vi "webqq.vi"(2 "获取好友列表按钮":bool, 3 "确定按钮":bool, 5 "退出登录按钮":bool, 6 "发送按钮":bool, 7 "要发送的内容":string, 10 "确认搜索按钮":bool, 11 "输入QQ昵称":string) -> (4 "发送返回值":string, 8 "获取好友标志":bool, 9 "搜索出的对应ID":string)   [LabVIEW 2016]
uses:
  <vilib>/httpClient/LabVIEWHTTPClient.lvlib
panel:
  out "链接标志":bool
  out "qqbat字符串":string
  out "昵称对应ID":string[](array[string])
  out "图片路径":path
  out "QQ昵称":string[](array[string])
  out "ID":i32[](array[numeric])
  out "数值":dbl
  out "error out 2":errorcluster caption="错误输出"
  out "好友列表字符串":string
  in  "id":string
  out "QQ登录二维码":picture
  out "路径 2":path
  out "error out":errorcluster caption="错误输出"
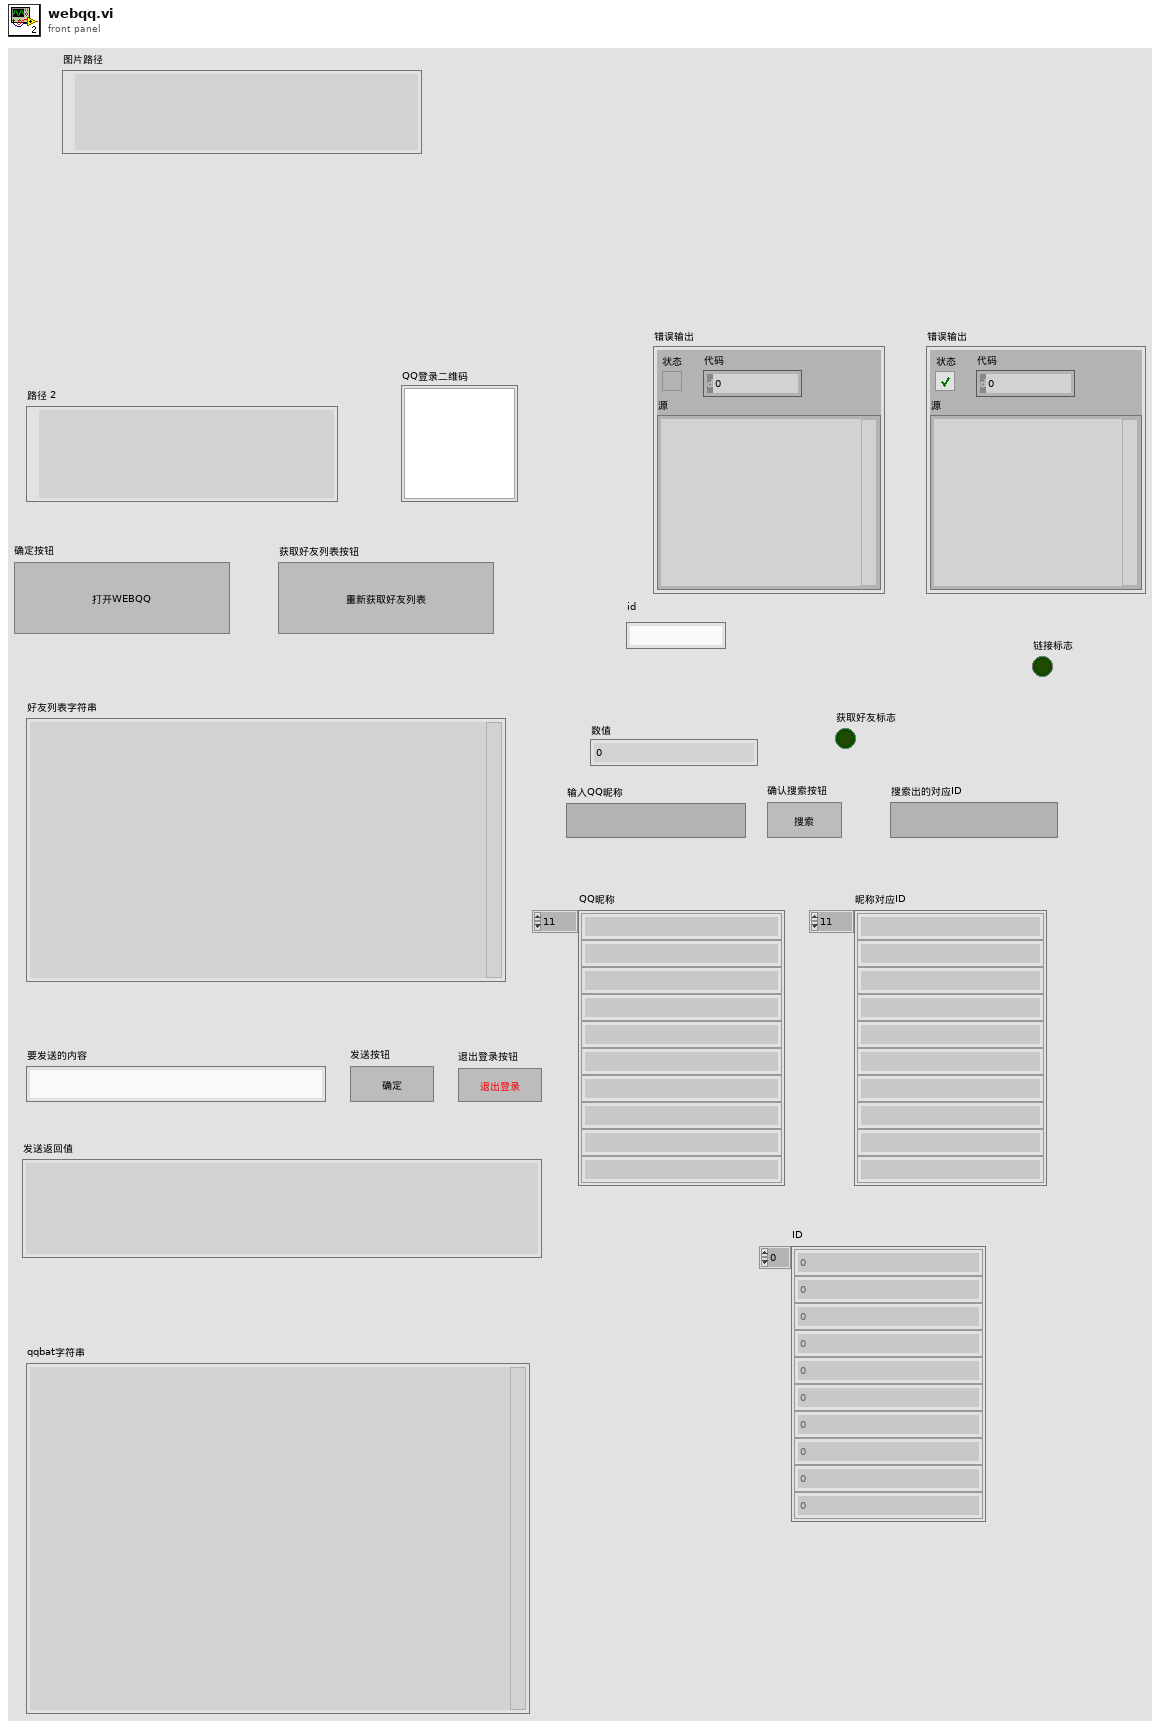
[diagram p1: front panel]
types:
  T1 = enum8{"Enabled", "Disabled", "Disabled and Grayed Out"}
  T2 = typedef "imagedata.ctl" = cluster{"image type":i32, "image depth":i32, "image":u8[], "mask":u8[], "colors":u32[], "Rectangle":cluster{"left":i16, "top":i16, "right":i16, "bottom":i16}}
  T3 = typedef "LabVIEWHTTPClient.lvlib/ClientHandle.ctl" = refnum<k1>
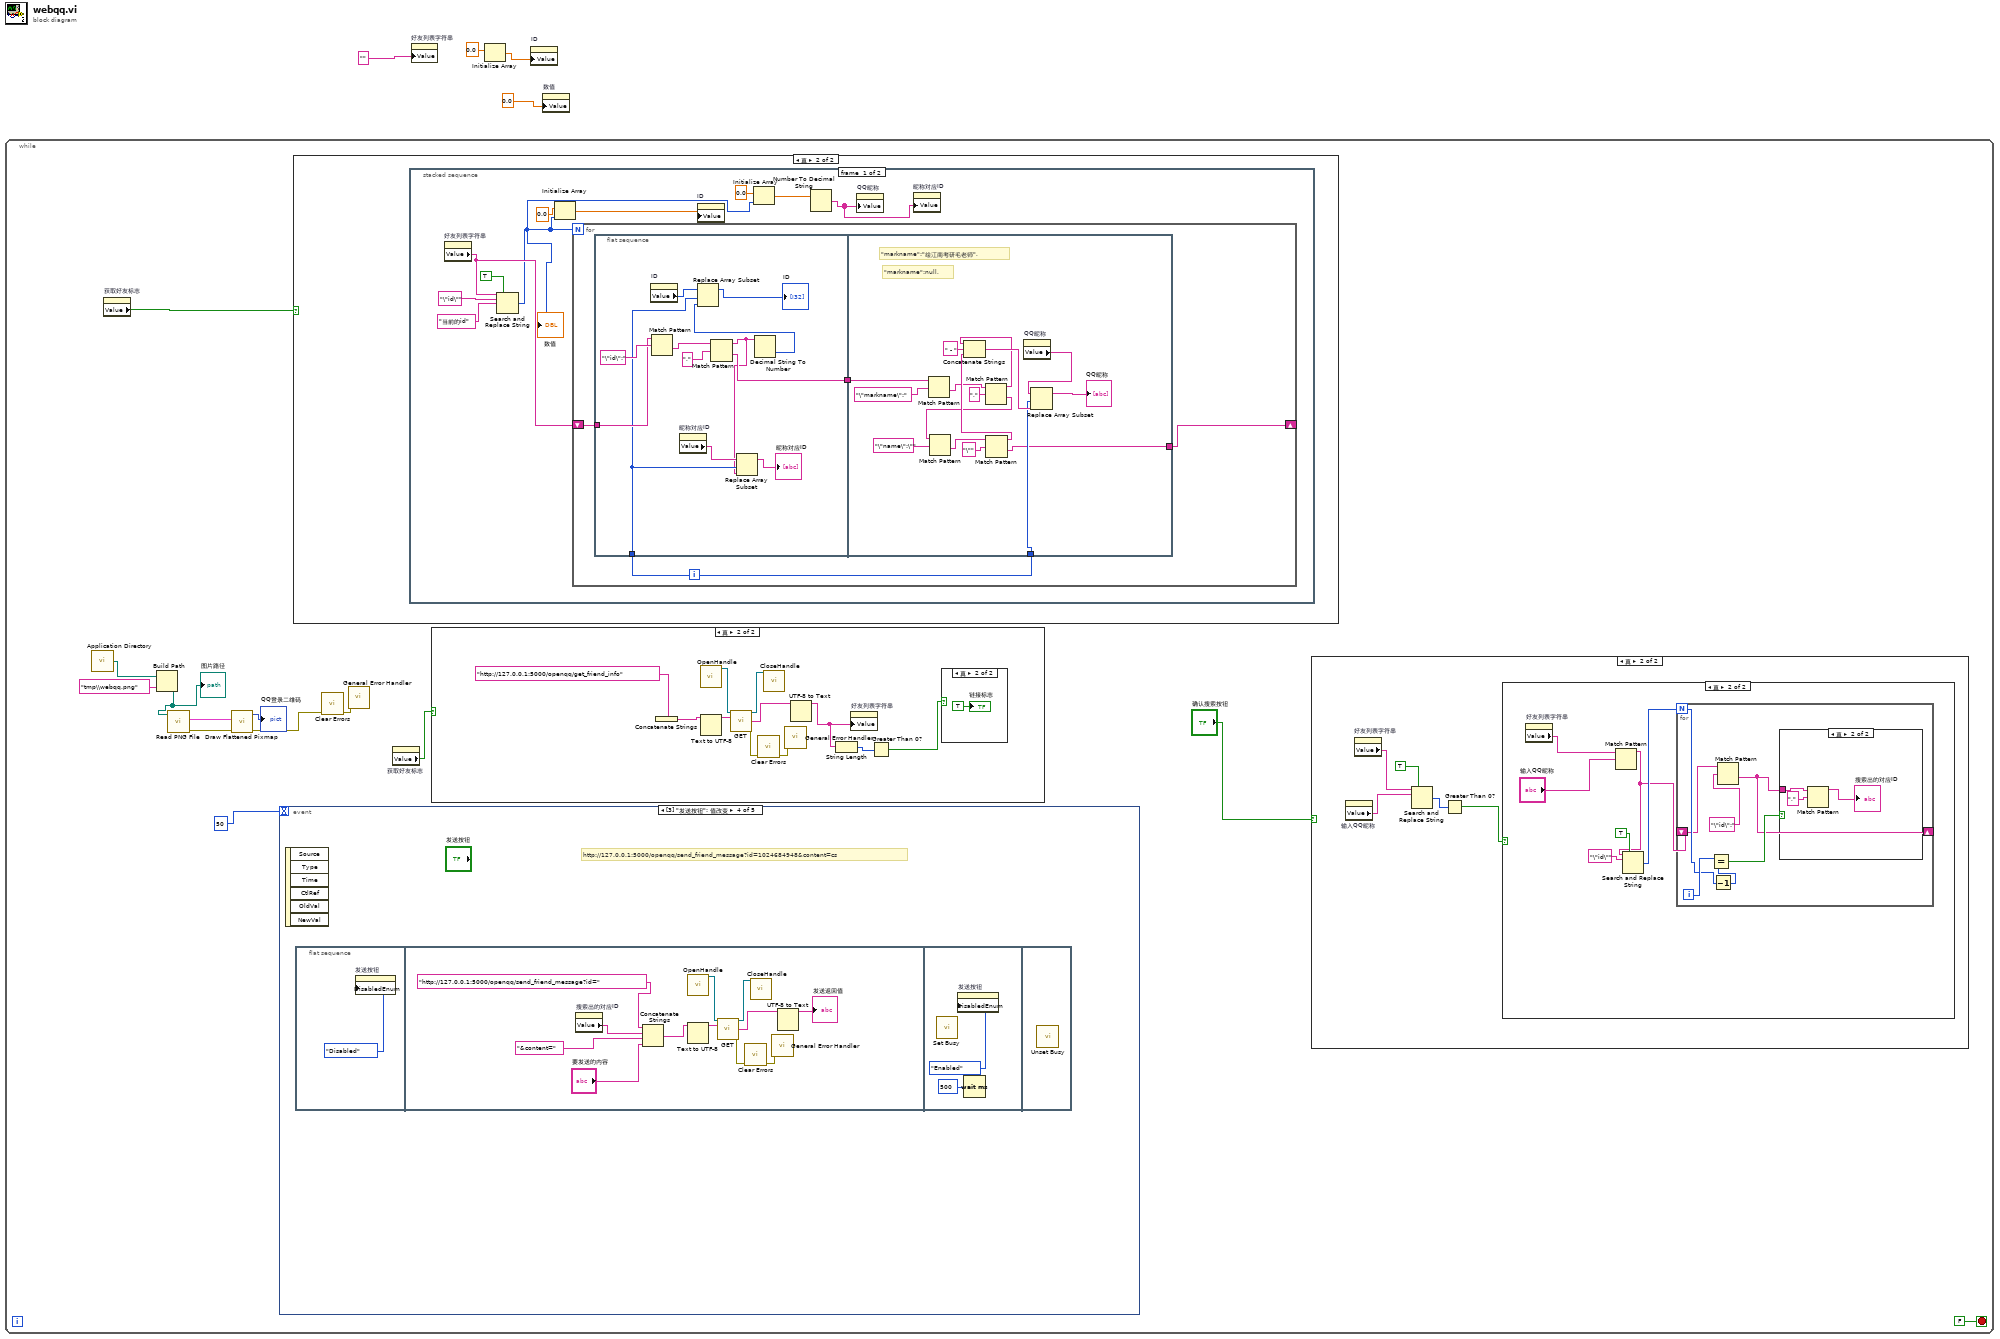
[diagram p0: block diagram]
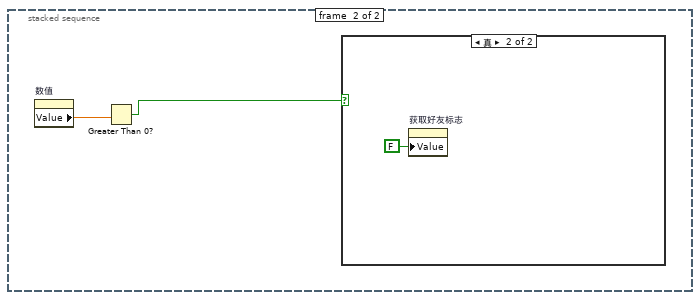
[diagram p8: hidden frame]
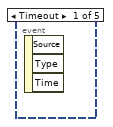
[diagram p10: hidden frame]
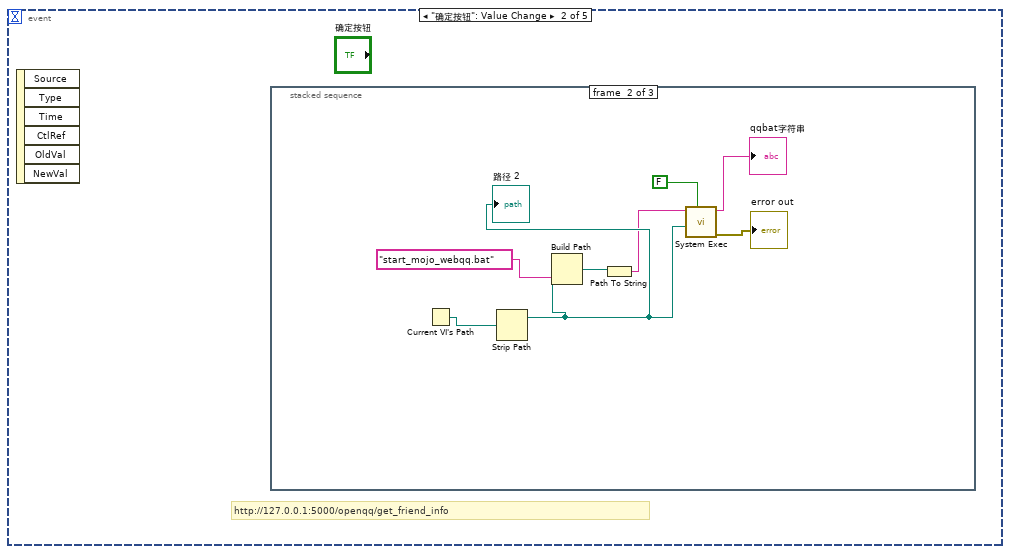
[diagram p11: hidden frame]
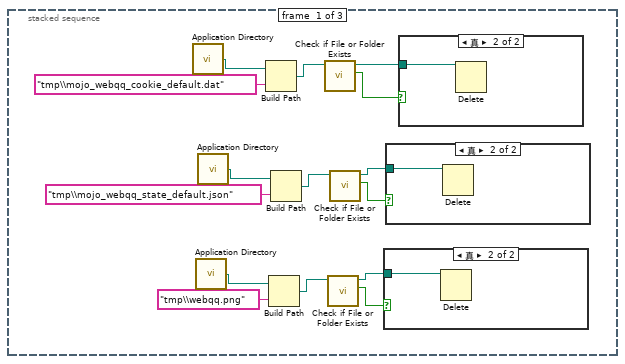
[diagram p12: hidden frame]
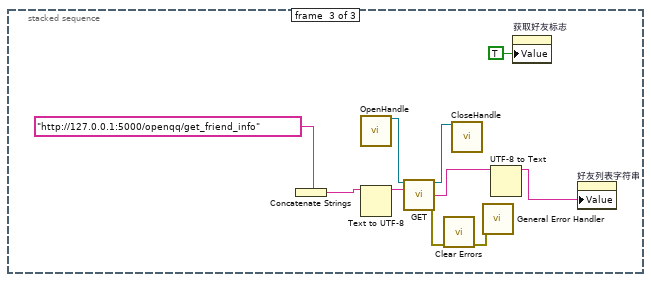
[diagram p16: hidden frame]
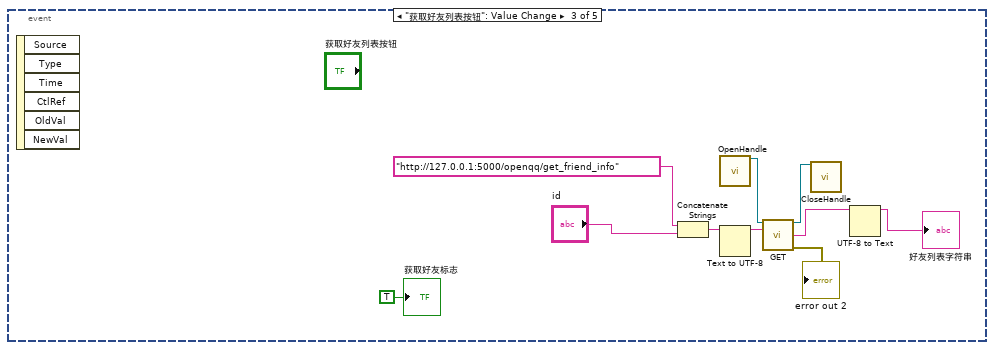
[diagram p17: hidden frame]
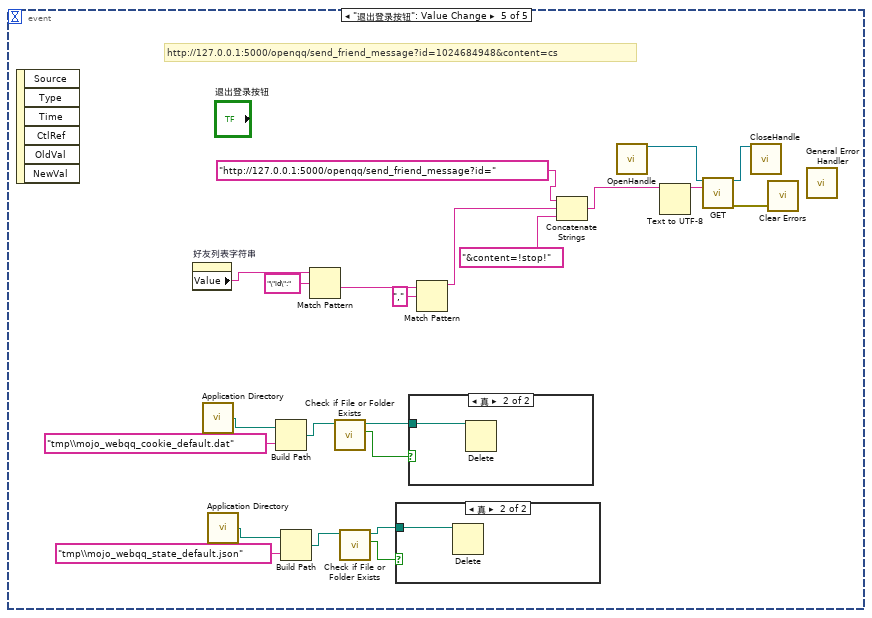
[diagram p18: hidden frame]
diagram:
  n1 = while {
    stop <- FALSE stop-if-true
    n2 = call <vilib>:"Application Directory.vi"() -> ("Application Directory"=w10:path)
    n3 = property on="获取好友标志" class="Bool (严格)"() -> ("Value"=w12:bool)  [unwired: 2 in, 2 out]
    n4 = Build Path(base path=w10, name or relative path="tmp\\webqq.png" ("名称或相对路径")) -> (appended path=w9:path)
    "图片路径" <- w9
    n5 = call <vilib>:"Read PNG File.vi"("path to PNG file"=w9) -> ("error out"=w5:errorcluster, "image data"=w16:T2)  [unwired: 8 in, 1 out]
    n6 = call <vilib>:"Draw Flattened Pixmap.vi"("image data"=w16) -> ("new picture"=→"QQ登录二维码":picture)  [unwired: 8 in]
    n7 = event shown="[3] \"发送按钮\": 值改变" {
      selector: _ -> [_ _ _ _ _]
      dyn-events: _ -> [_ _ _ _ _]
      timeout: 50 -> [_ _ _ _ _]
      event Timeout {
        n8 = event-data() -> ()  [unwired: 1 in, 3 out]
      }
      event "确定按钮": Value Change {
        # "http://127.0.0.1:5000/openqq/get_friend_info"
        n9 = event-data() -> ()  [unwired: 1 in, 6 out]
        n10 = stacked-sequence {
          frame #0 {
            n11 = call <vilib>:"Application Directory.vi"() -> ("Application Directory"=w100:path)
            n12 = call <vilib>:"Application Directory.vi"() -> ("Application Directory"=w97:path)
            n13 = call <vilib>:"Application Directory.vi"() -> ("Application Directory"=w107:path)
            n14 = Build Path(base path=w100, name or relative path="tmp\\mojo_webqq_cookie_default.dat" ("名称或相对路径")) -> (appended path=w102:path)
            n15 = Build Path(base path=w97, name or relative path="tmp\\webqq.png" ("名称或相对路径")) -> (appended path=w99:path)
            n16 = Build Path(base path=w107, name or relative path="tmp\\mojo_webqq_state_default.json" ("名称或相对路径")) -> (appended path=w105:path)
            n17 = call <vilib>:"Check if File or Folder Exists.vi"("path"=w102) -> ("file or folder exists?"=w103:bool, "dup path"=w104:path)  [unwired: 8 in, 1 out]
            n18 = call <vilib>:"Check if File or Folder Exists.vi"("path"=w99) -> ("file or folder exists?"=w96:bool, "dup path"=w95:path)  [unwired: 8 in, 1 out]
            n19 = call <vilib>:"Check if File or Folder Exists.vi"("path"=w105) -> ("file or folder exists?"=w108:bool, "dup path"=w109:path)  [unwired: 8 in, 1 out]
            n20 = case shown="真" w96 {
              tunnel: w95 -> [_ w110]
              frame False {
              }
              frame True {
                n21 = Delete(path (use dialog)=w110) -> ()  [unwired: 4 in, 3 out]
              }
            }
            n22 = case shown="真" w108 {
              tunnel: w109 -> [_ w111]
              frame False {
              }
              frame True {
                n23 = Delete(path (use dialog)=w111) -> ()  [unwired: 4 in, 3 out]
              }
            }
            n24 = case shown="真" w103 {
              tunnel: w104 -> [_ w112]
              frame False {
              }
              frame True {
                n25 = Delete(path (use dialog)=w112) -> ()  [unwired: 4 in, 3 out]
              }
            }
          }
          frame #1 {
            n26 = Current VI's Path() -> (path=w114:path)
            n27 = Strip Path(path=w114) -> (stripped path=w117:path)  [unwired: 1 out]
            "路径 2" <- w117
            n28 = Build Path(base path=w117, name or relative path="start_mojo_webqq.bat" ("名称或相对路径")) -> (appended path=w116:path)
            n29 = Path To String(path=w116) -> (string=w115:string)
            n30 = call <vilib>:"System Exec.vi"("wait until completion? (T)"=FALSE, "working directory"=w117, "command line"=w115) -> ("error out"=→"error out":errorcluster, "standard output"=→"qqbat字符串":string)  [unwired: 5 in, 2 out]
          }
          frame #2 {
            n31 = Concatenate Strings("http://127.0.0.1:5000/openqq/get_friend_info" ("字符串")) -> (w128:string)
            n32 = call <vilib>:"OpenHandle.vi"() -> ("client handle out"=w123:T3)  [unwired: 14 in, 1 out]
            n33 = Text to UTF-8(11:w128) -> (3:w126:string)  [unwired: 2 in, 1 out]
            n34 = call <vilib>:"GET.vi"("client handle"=w123, "url"=w126) -> ("client handle out"=w124:T3, "body"=w125:string, "error out"=w129:errorcluster)  [unwired: 10 in, 1 out]
            n35 = call <vilib>:"Clear Errors.vi"("error in (no error)"=w129) -> ("error out"=w130:errorcluster)  [unwired: 5 in, 1 out]
            n36 = call <vilib>:"CloseHandle.vi"("client handle"=w124) -> ()  [unwired: 14 in, 1 out]
            n37 = call <vilib>:"General Error Handler.vi"("error in (no error)"=w130) -> ()  [unwired: 10 in, 5 out]
            n38 = UTF-8 to Text(11:w125) -> (3:w121:string)  [unwired: 2 in, 1 out]
            n39 = property on="获取好友标志" class="Bool (严格)"("Value"=TRUE ("获取好友标志")) -> ()  [unwired: 2 in, 2 out]
            n40 = property on="好友列表字符串" class="Str"("Value"=w121) -> ()  [unwired: 2 in, 2 out]
          }
        }
      }
      event "获取好友列表按钮": Value Change {
        n41 = event-data() -> ()  [unwired: 1 in, 6 out]
        n42 = Concatenate Strings("http://127.0.0.1:5000/openqq/get_friend_info" ("字符串"), "id") -> (w139:string)
        n43 = call <vilib>:"OpenHandle.vi"() -> ("client handle out"=w134:T3)  [unwired: 14 in, 1 out]
        n44 = Text to UTF-8(11:w139) -> (3:w137:string)  [unwired: 2 in, 1 out]
        n45 = call <vilib>:"GET.vi"("client handle"=w134, "url"=w137) -> ("client handle out"=w135:T3, "body"=w136:string, "error out"=→"error out 2":errorcluster)  [unwired: 10 in, 1 out]
        n46 = call <vilib>:"CloseHandle.vi"("client handle"=w135) -> ()  [unwired: 14 in, 1 out]
        n47 = UTF-8 to Text(11:w136) -> (3:→"好友列表字符串":string)  [unwired: 2 in, 1 out]
        "获取好友标志" <- TRUE ("连接标志")
      }
      event "发送按钮": Value Change {
        # "http://127.0.0.1:5000/openqq/send_friend_message?id=1024684948&content=cs"
        n48 = event-data() -> ()  [unwired: 1 in, 6 out]
        n49 = flat-sequence {
          frame #0 {
            n50 = property on="发送按钮" class="Bool"("DisabledEnum"=T1."Disabled" ("禁用")) -> ()  [unwired: 2 in, 2 out]
          }
          frame #1 {
            n51 = property on="搜索出的对应ID" class="Str"() -> ("Value"=w144:string)  [unwired: 2 in, 2 out]
            n52 = Concatenate Strings("http://127.0.0.1:5000/openqq/send_friend_message?id=" ("字符串"), w144, "&content=" ("字符串"), "要发送的内容") -> (w151:string)
            n53 = call <vilib>:"OpenHandle.vi"() -> ("client handle out"=w146:T3)  [unwired: 14 in, 1 out]
            n54 = Text to UTF-8(11:w151) -> (3:w149:string)  [unwired: 2 in, 1 out]
            n55 = call <vilib>:"GET.vi"("client handle"=w146, "url"=w149) -> ("client handle out"=w147:T3, "body"=w148:string, "error out"=w152:errorcluster)  [unwired: 10 in, 1 out]
            n56 = call <vilib>:"Clear Errors.vi"("error in (no error)"=w152) -> ("error out"=w153:errorcluster)  [unwired: 5 in, 1 out]
            n57 = call <vilib>:"CloseHandle.vi"("client handle"=w147) -> ()  [unwired: 14 in, 1 out]
            n58 = call <vilib>:"General Error Handler.vi"("error in (no error)"=w153) -> ()  [unwired: 10 in, 5 out]
            n59 = UTF-8 to Text(11:w148) -> (3:→"发送返回值":string)  [unwired: 2 in, 1 out]
          }
          frame #2 {
            n60 = call <vilib>:"Set Busy.vi"() -> ()  [unwired: 10 in, 2 out]
            n61 = property on="发送按钮" class="Bool"("DisabledEnum"=T1."Enabled" ("禁用")) -> ()  [unwired: 2 in, 2 out]
            n62 = Wait (ms)(milliseconds to wait=u32 500 ("等待时间（毫秒）")) -> ()  [unwired: 1 out]
          }
          frame #3 {
            n63 = call <vilib>:"Unset Busy.vi"() -> ()  [unwired: 11 in, 1 out]
          }
        }
      }
      event "退出登录按钮": Value Change {
        # "http://127.0.0.1:5000/openqq/send_friend_message?id=1024684948&content=cs"
        n64 = event-data() -> ()  [unwired: 1 in, 6 out]
        n65 = property on="好友列表字符串" class="Str"() -> ("Value"=w161:string)  [unwired: 2 in, 2 out]
        n66 = call <vilib>:"Application Directory.vi"() -> ("Application Directory"=w177:path)
        n67 = call <vilib>:"Application Directory.vi"() -> ("Application Directory"=w170:path)
        n68 = Build Path(base path=w177, name or relative path="tmp\\mojo_webqq_cookie_default.dat" ("名称或相对路径")) -> (appended path=w175:path)
        n69 = Build Path(base path=w170, name or relative path="tmp\\mojo_webqq_state_default.json" ("名称或相对路径")) -> (appended path=w172:path)
        n70 = Match Pattern(string=w161, regular expression="\"id\":" ("正则表达式")) -> (after substring=w159:string)  [unwired: 1 in, 3 out]
        n71 = call <vilib>:"Check if File or Folder Exists.vi"("path"=w175) -> ("file or folder exists?"=w174:bool, "dup path"=w173:path)  [unwired: 8 in, 1 out]
        n72 = call <vilib>:"Check if File or Folder Exists.vi"("path"=w172) -> ("file or folder exists?"=w169:bool, "dup path"=w168:path)  [unwired: 8 in, 1 out]
        n73 = case shown="真" w169 {
          tunnel: w168 -> [_ w178]
          frame False {
          }
          frame True {
            n74 = Delete(path (use dialog)=w178) -> ()  [unwired: 4 in, 3 out]
          }
        }
        n75 = case shown="真" w174 {
          tunnel: w173 -> [_ w179]
          frame False {
          }
          frame True {
            n76 = Delete(path (use dialog)=w179) -> ()  [unwired: 4 in, 3 out]
          }
        }
        n77 = Match Pattern(string=w159, regular expression="," ("正则表达式")) -> (before substring=w157:string)  [unwired: 1 in, 3 out]
        n78 = Concatenate Strings("http://127.0.0.1:5000/openqq/send_friend_message?id=" ("字符串"), w157, "&content=!stop!" ("字符串")) -> (w162:string)
        n79 = call <vilib>:"OpenHandle.vi"() -> ("client handle out"=w165:T3)  [unwired: 14 in, 1 out]
        n80 = Text to UTF-8(11:w162) -> (3:w167:string)  [unwired: 2 in, 1 out]
        n81 = call <vilib>:"GET.vi"("client handle"=w165, "url"=w167) -> ("client handle out"=w164:T3, "error out"=w166:errorcluster)  [unwired: 10 in, 2 out]
        n82 = call <vilib>:"CloseHandle.vi"("client handle"=w164) -> ()  [unwired: 14 in, 1 out]
        n83 = call <vilib>:"Clear Errors.vi"("error in (no error)"=w166) -> ()  [unwired: 5 in, 2 out]
        n84 = call <vilib>:"General Error Handler.vi"() -> ()  [unwired: 11 in, 5 out]
      }
    }
    n85 = case shown="真" w12 {
      frame False {
      }
      frame True {
        n86 = stacked-sequence {
          frame #0 {
            n87 = property on="好友列表字符串" class="Str"() -> ("Value"=w56:string)  [unwired: 2 in, 2 out]
            n88 = Search and Replace String(replace all?=TRUE ("替换全部？(F)"), input string=w56, search string="\"id\"" ("搜索字符串"), replace string="当前的id" ("替换字符串(\"\")")) -> (number of replacements=w52:i32)  [unwired: 4 in, 3 out]
            "数值" <- w52
            n89 = Initialize Array(0.0 ("元素"), w52) -> (w54:dbl[])
            n90 = for {
              N: w52 -> [_]
              shift-right: [w61] -> _
              shift-left: w56 -> [w63]
              i -> [w62]
              n91 = flat-sequence {
                tunnel: w63 -> [w69]
                tunnel: w62 -> [w66]
                tunnel: [w68] -> w60
                tunnel: w62 -> [w80]
                tunnel: [w79] -> w61
                tunnel: w60 -> [w78]
                frame #0 {
                  n92 = property on="ID" class="Arr (严格)"() -> ("Value"=w72:i32[])  [unwired: 2 in, 2 out]
                  n93 = Match Pattern(string=w69, regular expression="\"id\":" ("正则表达式")) -> (after substring=w74:string)  [unwired: 1 in, 3 out]
                  n94 = property on="昵称对应ID" class="Arr (严格)"() -> ("Value"=w67:string[])  [unwired: 2 in, 2 out]
                  n95 = Match Pattern(string=w74, regular expression="," ("正则表达式")) -> (before substring=w65:string, after substring=w68:string)  [unwired: 1 in, 2 out]
                  n96 = Replace Array Subset(array=w67, new element=w65, index=w66) -> (→"昵称对应ID":string[])
                  n97 = Decimal String To Number(string=w65) -> (number=w71:i32)  [unwired: 2 in, 1 out]
                  n98 = Replace Array Subset(array=w72, new element=w71, index=w66) -> (→"ID":i32[])
                }
                frame #1 {
                  # "\"markname\":null,"
                  # "\"markname\":\"绘江南考研毛老师\","
                  n99 = Match Pattern(string=w78, regular expression="\"markname\":" ("正则表达式")) -> (after substring=w82:string)  [unwired: 1 in, 3 out]
                  n100 = Match Pattern(string=w82, regular expression="," ("正则表达式")) -> (before substring=w76:string, after substring=w77:string)  [unwired: 1 in, 2 out]
                  n101 = Match Pattern(string=w77, regular expression="\"name\":\"" ("正则表达式")) -> (after substring=w89:string)  [unwired: 1 in, 3 out]
                  n102 = Match Pattern(string=w89, regular expression="\"" ("正则表达式")) -> (before substring=w91:string, after substring=w79:string)  [unwired: 1 in, 2 out]
                  n103 = Concatenate Strings(w76, " - " ("字符串"), w91) -> (w90:string)
                  n104 = property on="QQ昵称" class="Arr (严格)"() -> ("Value"=w84:string[])  [unwired: 2 in, 2 out]
                  n105 = Replace Array Subset(array=w84, new element=w90, index=w80) -> (→"QQ昵称":string[])
                }
              }
            }
            n106 = property on="ID" class="Arr (严格)"("Value"=w54) -> ()  [unwired: 2 in, 2 out]
            n107 = Initialize Array(0.0 ("元素"), w52) -> (w51:dbl[])
            n108 = Number To Decimal String(number=w51) -> (decimal integer string=w50:string[])  [unwired: 1 in]
            n109 = property on="QQ昵称" class="Arr (严格)"("Value"=w50) -> ()  [unwired: 2 in, 2 out]
            n110 = property on="昵称对应ID" class="Arr (严格)"("Value"=w50) -> ()  [unwired: 2 in, 2 out]
          }
          frame #1 {
            n111 = property on="数值" class="DigNum (严格)"() -> ("Value"=w93:dbl)  [unwired: 2 in, 2 out]
            n112 = Greater Than 0?(x=w93) -> (x > 0?=w92:bool)
            n113 = case shown="真" w92 {
              frame False {
              }
              frame True {
                n114 = property on="获取好友标志" class="Bool (严格)"("Value"=FALSE ("连接标志")) -> ()  [unwired: 2 in, 2 out]
              }
            }
          }
        }
      }
    }
    n115 = call <vilib>:"Clear Errors.vi"("error in (no error)"=w5) -> ("error out"=w6:errorcluster)  [unwired: 5 in, 1 out]
    n116 = call <vilib>:"General Error Handler.vi"("error in (no error)"=w6) -> ()  [unwired: 10 in, 5 out]
    n117 = property on="获取好友标志" class="Bool (严格)"() -> ("Value"=w7:bool)  [unwired: 2 in, 2 out]
    n118 = case shown="真" w7 {
      frame False {
      }
      frame True {
        n119 = Concatenate Strings("http://127.0.0.1:5000/openqq/get_friend_info" ("字符串")) -> (w22:string)
        n120 = call <vilib>:"OpenHandle.vi"() -> ("client handle out"=w27:T3)  [unwired: 14 in, 1 out]
        n121 = Text to UTF-8(11:w22) -> (3:w24:string)  [unwired: 2 in, 1 out]
        n122 = call <vilib>:"GET.vi"("client handle"=w27, "url"=w24) -> ("client handle out"=w26:T3, "body"=w25:string, "error out"=w21:errorcluster)  [unwired: 10 in, 1 out]
        n123 = call <vilib>:"Clear Errors.vi"("error in (no error)"=w21) -> ("error out"=w20:errorcluster)  [unwired: 5 in, 1 out]
        n124 = call <vilib>:"CloseHandle.vi"("client handle"=w26) -> ()  [unwired: 14 in, 1 out]
        n125 = call <vilib>:"General Error Handler.vi"("error in (no error)"=w20) -> ()  [unwired: 10 in, 5 out]
        n126 = UTF-8 to Text(11:w25) -> (3:w19:string)  [unwired: 2 in, 1 out]
        n127 = String Length(string=w19) -> (length=w18:i32)
        n128 = property on="好友列表字符串" class="Str"("Value"=w19) -> ()  [unwired: 2 in, 2 out]
        n129 = Greater Than 0?(x=w18) -> (x > 0?=w17:bool)
        n130 = case shown="真" w17 {
          frame False {
          }
          frame True {
            "链接标志" <- TRUE ("链接标志")
          }
        }
      }
    }
    n131 = case shown="真" "确认搜索按钮" {
      frame False {
      }
      frame True {
        n132 = property on="输入QQ昵称" class="Str"() -> ("Value"=w32:string)  [unwired: 2 in, 2 out]
        n133 = property on="好友列表字符串" class="Str"() -> ("Value"=w33:string)  [unwired: 2 in, 2 out]
        n134 = Search and Replace String(replace all?=TRUE ("替换全部？(F)"), input string=w33, search string=w32) -> (number of replacements=w30:i32)  [unwired: 5 in, 3 out]
        n135 = Greater Than 0?(x=w30) -> (x > 0?=w29:bool)
        n136 = case shown="真" w29 {
          frame False {
          }
          frame True {
            n137 = property on="好友列表字符串" class="Str"() -> ("Value"=w39:string)  [unwired: 2 in, 2 out]
            n138 = Match Pattern(string=w39, regular expression="输入QQ昵称") -> (before substring=w35:string)  [unwired: 1 in, 3 out]
            n139 = Search and Replace String(replace all?=TRUE ("替换全部？(F)"), input string=w35, search string="\"id\"" ("搜索字符串")) -> (number of replacements=w36:i32)  [unwired: 5 in, 3 out]
            n140 = for {
              N: w36 -> [w43]
              shift-right: [w40] -> _
              shift-left: w35 -> [w41]
              i -> [w45]
              n141 = Decrement(x=w43) -> (x-1=w42:i32)
              n142 = Equal?(x=w45, y=w42) -> (x = y?=w44:bool)
              n143 = Match Pattern(string=w41, regular expression="\"id\":" ("正则表达式")) -> (after substring=w40:string)  [unwired: 1 in, 3 out]
              n144 = case shown="真" w44 {
                tunnel: w40 -> [_ w48]
                frame False {
                }
                frame True {
                  n145 = Match Pattern(string=w48, regular expression="," ("正则表达式")) -> (before substring=→"搜索出的对应ID":string)  [unwired: 1 in, 3 out]
                }
              }
            }
          }
        }
      }
    }
  }
  n146 = property on="好友列表字符串" class="Str"("Value"="" ("字符串")) -> ()  [unwired: 2 in, 2 out]
  n147 = Initialize Array(0.0 ("元素")) -> (w3:dbl[])  [unwired: 1 in]
  n148 = property on="ID" class="Arr (严格)"("Value"=w3) -> ()  [unwired: 2 in, 2 out]
  n149 = property on="数值" class="DigNum (严格)"("Value"=0.0 ("数值 2")) -> ()  [unwired: 2 in, 2 out]
